vi "Pcre2GetMatchOffsetsFromMatchData8.vi"(8 "error in":errorcluster, 11 "pMatchData":u64 format="%.0x") -> (0 "error out":errorcluster, 1 "OffsetsPastMatch":i32[](array[numeric]), 2 "MatchOffsets":i32[](array[numeric]), 3 "pMatchData":u64 format="%.0x")   [LabVIEW 2021, in "libpcre2-8.lvlib"]
uses:
  libpcre2-8.lvlib
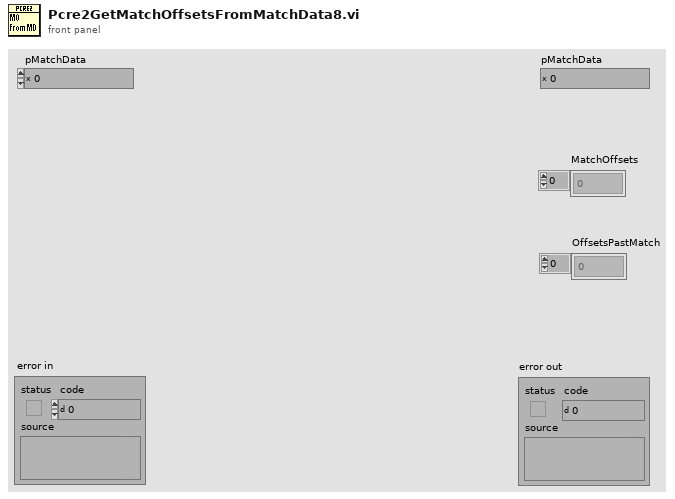
[diagram p1: front panel]
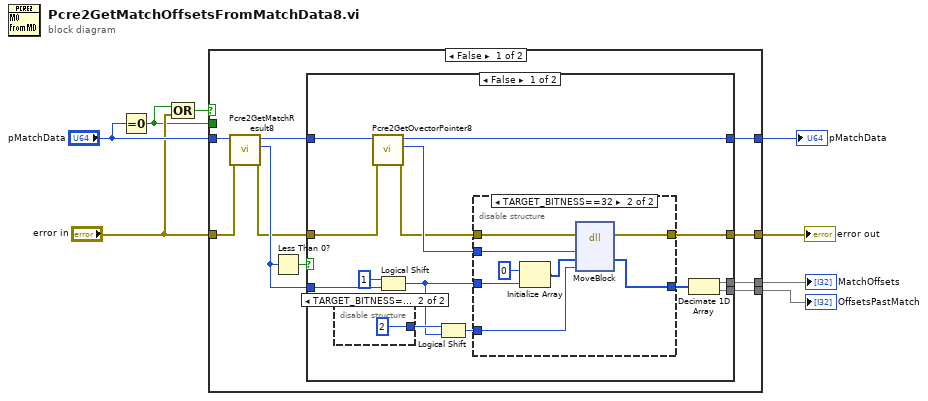
[diagram p0: block diagram]
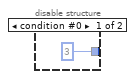
[diagram p2: hidden frame]
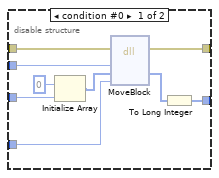
[diagram p3: hidden frame]
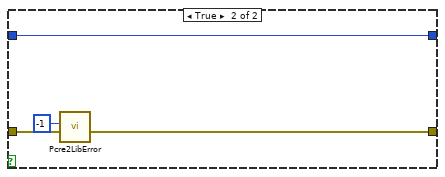
[diagram p4: hidden frame]
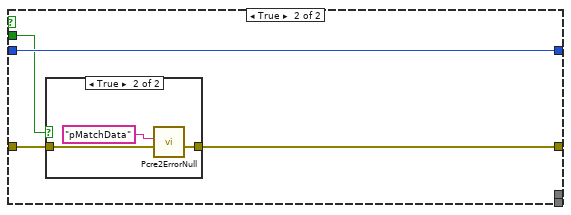
[diagram p5: hidden frame]
diagram:
  n1 = Equal To 0?(x="pMatchData") -> (x = 0?=w1:bool)
  n2 = Compound Arithmetic op=OR(w1, "error in") -> (w3:bool)
  n3 = case shown="False" w3 {
    tunnel: "error in" -> [w9 w56]
    tunnel: [w18 w58] -> w8
    tunnel: "pMatchData" -> [w14 w59]
    tunnel: [w15 w59] -> w7
    tunnel: [w17 _] -> w5
    tunnel: [w16 _] -> w4
    tunnel: w1 -> [_ w57]
    frame False {
      n4 = call "Pcre2GetMatchResult8.vi"("error in"=w9, "pMatchData"=w14) -> ("error out"=w10:errorcluster, "MatchResult"=w13:i32, "pMatchData"=w11:u64)  [unwired: 7 in]
      n5 = Less Than 0?(x=w13) -> (x < 0?=w12:bool)
      n6 = case shown="False" w12 {
        tunnel: [w32 w53] -> w18
        tunnel: [w30 _] -> w17
        tunnel: [w29 _] -> w16
        tunnel: [w23 w52] -> w15
        tunnel: w10 -> [w19 w54]
        tunnel: w11 -> [w21 w52]
        tunnel: w13 -> [w22 _]
        frame False {
          n7 = disable-structure shown="TARGET_BITNESS==32" {
            disable-tunnel: [i16 3 ("y") i16 2 ("y")] -> w25
            frame condition #0 {
            }
            frame condition #1 (active) {
            }
          }
          n8 = call "Pcre2GetOvectorPointer8.vi"("error in"=w19, "pMatchData"=w21) -> ("error out"=w20:errorcluster, "pOvector"=w28:u64, "pMatchData"=w23:u64)  [unwired: 7 in]
          n9 = Logical Shift(y=i16 1, x=w22) -> (x << y=w24:i32)
          n10 = Logical Shift(y=w25, x=w24) -> (x << y=w26:i32)
          n11 = disable-structure shown="TARGET_BITNESS==32" {
            disable-tunnel: w28 -> [w43 w51]
            disable-tunnel: [w42 w50] -> w32
            disable-tunnel: w20 -> [w41 w49]
            disable-tunnel: w26 -> [w39 w47]
            disable-tunnel: w24 -> [w38 w46]
            disable-tunnel: [w35 w44] -> w31
            frame condition #0 {
              n12 = Initialize Array(i64 0 ("element"), w38) -> (w37:i64[])
              n13 = dll-call lib="LabVIEW" fn="MoveBlock"(error in=w41, "pointerSrc"=w43, "pointerDest"=w37, "size"=w39) -> (error out=w42:errorcluster, "pointerDest"=w36:i64[])  [unwired: 5 in, 1 out]
              n14 = To Long Integer(number=w36) -> (32bit integer=w35:i32[])
            }
            frame condition #1 (active) {
              n15 = Initialize Array(0 ("element"), w46) -> (w45:i32[])
              n16 = dll-call lib="LabVIEW" fn="MoveBlock"(error in=w49, "pointerSrc"=w51, "pointerDest"=w45, "size"=w47) -> (error out=w50:errorcluster, "pointerDest"=w44:i32[])  [unwired: 5 in, 1 out]
            }
          }
          n17 = Decimate 1D Array(w31) -> (w30:i32[], w29:i32[])
        }
        frame True {
          n18 = call "Pcre2LibError.vi"("error in"=w54, "ErrorCode"=-1) -> ("error out"=w53:errorcluster)  [unwired: 9 in]
        }
      }
    }
    frame True {
      n19 = case shown="True" w57 {
        tunnel: w56 -> [w60 w62]
        tunnel: [w60 w61] -> w58
        frame False {
        }
        frame True {
          n20 = call "Pcre2ErrorNull.vi"("error in"=w62, "What"="pMatchData") -> ("error out"=w61:errorcluster)  [unwired: 9 in]
        }
      }
    }
  }
  "pMatchData" <- w7
  "error out" <- w8
  "MatchOffsets" <- w5
  "OffsetsPastMatch" <- w4
